vi "Substitute Actor.vi"(10 "Substitute Actor in":refnum<class "Actor.lvclass">, 11 "Current Monitored Actor":refnum<class "Monitored Actor.lvclass">) -> (0 "error out":errorcluster, 2 "Substitute Actor out":refnum<class "Actor.lvclass">)   [LabVIEW 2017, in "MGI-Monitored Actor Core.lvlib" / "Monitored Actor.lvclass"]
doc: "(<B>Filename</B>: Actor Framework.lvlib:Actor.lvclass:Substitute Actor.vi)\n\nThis method copies information from the <b>Current Actor</b> to the <b>Substitute Actor</b>, including the to-self and the to-caller queue references. The purpose of this function is to allow an actor to define a method that replaces itself with another actor, useful for implementing a State Pattern Actor. Child classes should override this method to copy any additional fields that they need from the current to the substitute.\n\nThis method may return error code 678010: Illegal substitution. Overrides of this method may choose to return this error if the new actor is not one that is an appropriate substitute for the current actor, for whatever standards of \"appropriate\" are chosen for the current actor. If returning an error, override VIs should return the unmodified <b>Current Actor</b> as <b>Substitute Actor out</b>."
uses:
  Monitored Actor.lvclass
  C:/Program Files (x86)/National Instruments/LabVIEW 2017/vi.lib/ActorFramework/Actor/Actor.lvclass
  <vilib>/ActorFramework/Actor/Actor.lvclass
  Monitored Actor.lvclass/Monitored Actor.ctl
  <vilib>/ActorFramework/Actor/Actor.lvclass/Actor.ctl
  <vilib>/ActorFramework/Message Enqueuer/Message Enqueuer.lvclass/Message Enqueuer.ctl
  <vilib>/ActorFramework/Message Enqueuer/Init from Existing Queue.vi
  <vilib>/ActorFramework/Message Enqueuer/Message Enqueuer.lvclass
  Actor Monitor/Actor Monitor Messages/Actor Stopped Msg/Actor Stopped Msg.lvclass
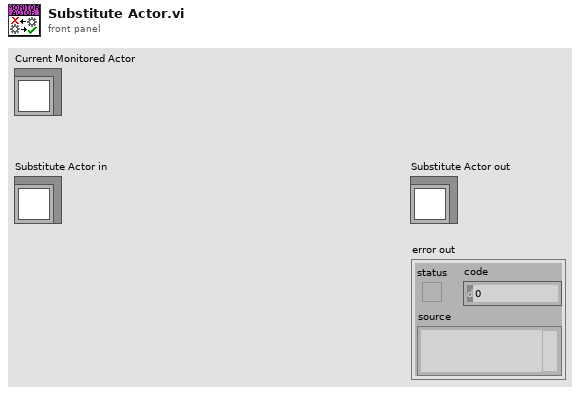
[diagram p1: front panel]
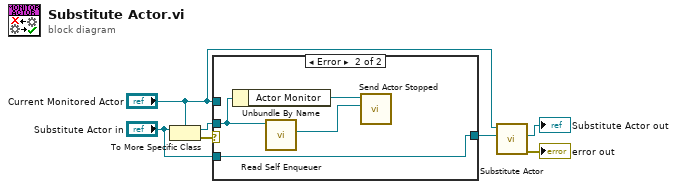
[diagram p0: block diagram]
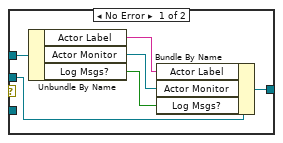
[diagram p2: hidden frame]
diagram:
  n1 = To More Specific Class(target class="Current Monitored Actor", reference="Substitute Actor in") -> (specific class reference=w4:refnum<class "Monitored Actor.lvclass">, error out=w2:errorcluster)  [unwired: 1 in]
  n2 = case shown="Error" w2 {
    tunnel: "Current Monitored Actor" -> [w13 _]
    tunnel: w4 -> [w12 w15]
    tunnel: [w11 w14] -> w3
    tunnel: "Substitute Actor in" -> [_ w14]
    frame No Error {
      n3 = Unbundle By Name(w13) -> ("Actor Label"=w10:string, "Actor Monitor"=w9:refnum<class "Message Enqueuer.lvclass">, "Log Msgs?"=w8:bool)
      n4 = Bundle By Name(cluster=w12, "Actor Label"=w10, "Actor Monitor"=w9, "Log Msgs?"=w8) -> (w11:refnum<class "Monitored Actor.lvclass">)
    }
    frame Error {
      n5 = Unbundle By Name(w15) -> ("Actor Monitor"=w16:refnum<class "Message Enqueuer.lvclass">)
      n6 = call <vilib>:"Read Self Enqueuer.vi"("Actor"=w15) -> ("Self Enqueuer"=w17:refnum<class "Message Enqueuer.lvclass">)  [unwired: 10 in]
      n7 = call "Send Actor Stopped.vi"("Actor's Self Q"=w17, "Message Enqueuer in"=w16) -> ()  [unwired: 8 in, 2 out]
    }
  }
  n8 = call-parent "Substitute Actor.vi"("Substitute Actor in"=w3, "Current Actor"="Current Monitored Actor") -> ("error out"=→"error out":errorcluster, "Substitute Actor out"=→"Substitute Actor out":refnum<class "Actor.lvclass">)  [unwired: 8 in]
